vi "Corr_stats_labels.vi"(2 "Inst 2 Units":T1={"Colour"=0, "Inst type"=enum."Pitot-static tube", "Inst name"="Manometer voltage", "Symbol"="U", "Code name"="", "Extra Info"="U", "Inst Array"=enum."PWA", "Index"=0, "Voltage Index"=0, "Extra Titles"=[], "Extra Values"=[]}, 3 "Inst 1 Units":T1={"Colour"=0, "Inst type"=enum."Pitot-static tube", "Inst name"="Manometer voltage", "Symbol"="U", "Code name"="", "Extra Info"="U", "Inst Array"=enum."PWA", "Index"=0, "Voltage Index"=0, "Extra Titles"=[], "Extra Values"=[]}) -> (0 "Output":string[](array[string]))   [LabVIEW 2010]
uses:
  Controls/Analysis_info_cluster.ctl
  Controls/Inst_type.ctl
  Controls/Instrument_Array.ctl
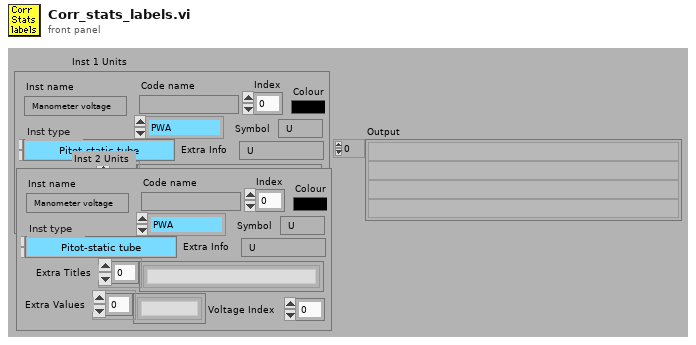
[diagram p1: front panel]
types:
  T1 = typedef "Analysis_info_cluster.ctl" = cluster{"Colour":u32, "Inst type":T2, "Inst name":string, "Symbol":string, "Code name":string, "Extra Info":string, "Inst Array":T3, "Index":i32, "Voltage Index":i32, "Extra Titles":string[], "Extra Values":string[]}
  T2 = typedef "Inst_type.ctl" = enum16{"Propeller anemometer", "Raw voltage", "Pressure Transducer", "Pitot-static tube", "Preston tube", "Hot wire", "Cross wire 1", "Cross wire 2", "Generic Linear", "Generic Polynomial", "Generic BackPoly", "Fast FID", "Thermocouple", "Cold wire", "Pulsed Wire", "LDA Vel", "LDA Tran time", "LDA Arr time"}
  T3 = typedef "Instrument_Array.ctl" = enum16{"PWA", "LDA", "Analogue"}
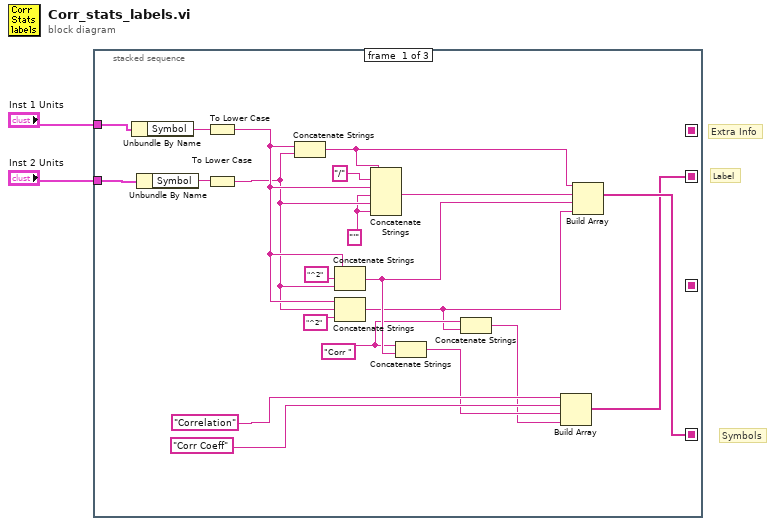
[diagram p0: block diagram]
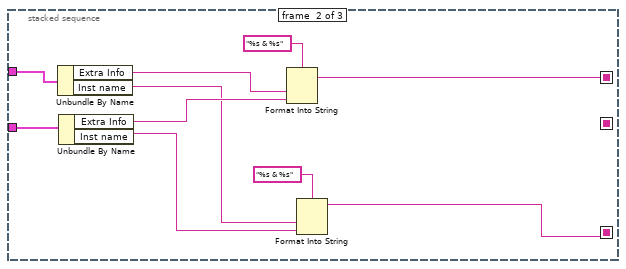
[diagram p2: hidden frame]
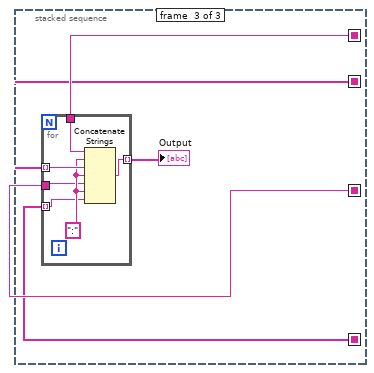
[diagram p3: hidden frame]
diagram:
  # "Extra Info"
  # "Label"
  # "Symbols"
  n1 = stacked-sequence {
    seq-local: [w15 _ _] -> [_ _ w35]
    seq-local: [w14 _ _] -> [_ _ w37]
    seq-local: [_ w25 _] -> [_ _ w38]
    seq-local: [_ w24 _] -> [_ _ w36]
    tunnel: "Inst 2 Units" -> [w19 w32 _]
    tunnel: "Inst 1 Units" -> [w16 w33 _]
    frame #0 {
      w5 = "Corr "
      w9 = "'"
      n2 = Unbundle By Name(w16) -> ("Symbol"=w18:string)
      n3 = Unbundle By Name(w19) -> ("Symbol"=w17:string)
      n4 = To Lower Case(string=w18) -> (all lower case string=w23:string)
      n5 = To Lower Case(string=w17) -> (all lower case string=w22:string)
      n6 = Concatenate Strings(w23, w22) -> (w11:string)
      n7 = Concatenate Strings(w23, "^2", w22) -> (w7:string)
      n8 = Concatenate Strings(w23, w22, "^2") -> (w4:string)
      n9 = Concatenate Strings(w11, "/", w23, w9, w22, w9) -> (w8:string)
      n10 = Concatenate Strings(w5, w7) -> (w6:string)
      n11 = Concatenate Strings(w5, w4) -> (w3:string)
      n12 = Build Array("Correlation", "Corr Coeff", w6, w3) -> (w14:string[])
      n13 = Build Array(w11, w8, w7, w4) -> (w15:string[])
    }
    frame #1 {
      n14 = Unbundle By Name(w33) -> ("Extra Info"=w31:string, "Inst name"=w27:string)
      n15 = Unbundle By Name(w32) -> ("Extra Info"=w30:string, "Inst name"=w26:string)
      n16 = Format Into String(format string="%s & %s" ("Format String"), w31, w30) -> (resulting string=w25:string)  [unwired: 2 in, 1 out]
      n17 = Format Into String(format string="%s & %s" ("Format String"), w27, w26) -> (resulting string=w24:string)  [unwired: 2 in, 1 out]
    }
    frame #2 {
      n18 = for {
        tunnel: [w44] -> w34 mode=indexing
        tunnel: w38 -> [w43]
        tunnel: w37 -> [w42] mode=indexing
        tunnel: w36 -> [w40]
        tunnel: w35 -> [w39] mode=indexing
        w41 = ":" ("Substring")
        n19 = Concatenate Strings(w43, w41, w42, w41, w40, w41, w39) -> (w44:string)
      }
      "Output" <- w34
    }
  }
